vi "Check Status.vi"(8 "error in (no error)":errorcluster, 11 "Power Meter in":refnum<class "Power Meter.lvclass">) -> (0 "error out":errorcluster, 1 "Status":string, 2 "Ready?":bool, 3 "Power Meter out":refnum<class "Power Meter.lvclass">)   [LabVIEW 2009, in "Power Meter.lvclass"]
doc: "(Dynamic) Check if the instrument is powered on and update its member fields with the instrument's current status. Optionally return a text status message."
uses:
  Power Meter.lvclass
  Utility Classes/Readable/Readable.lvclass
  Power Meter.lvclass/Power Meter.ctl
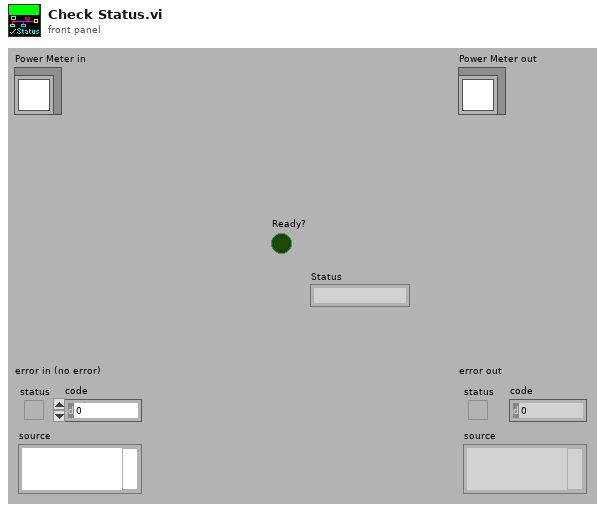
[diagram p1: front panel]
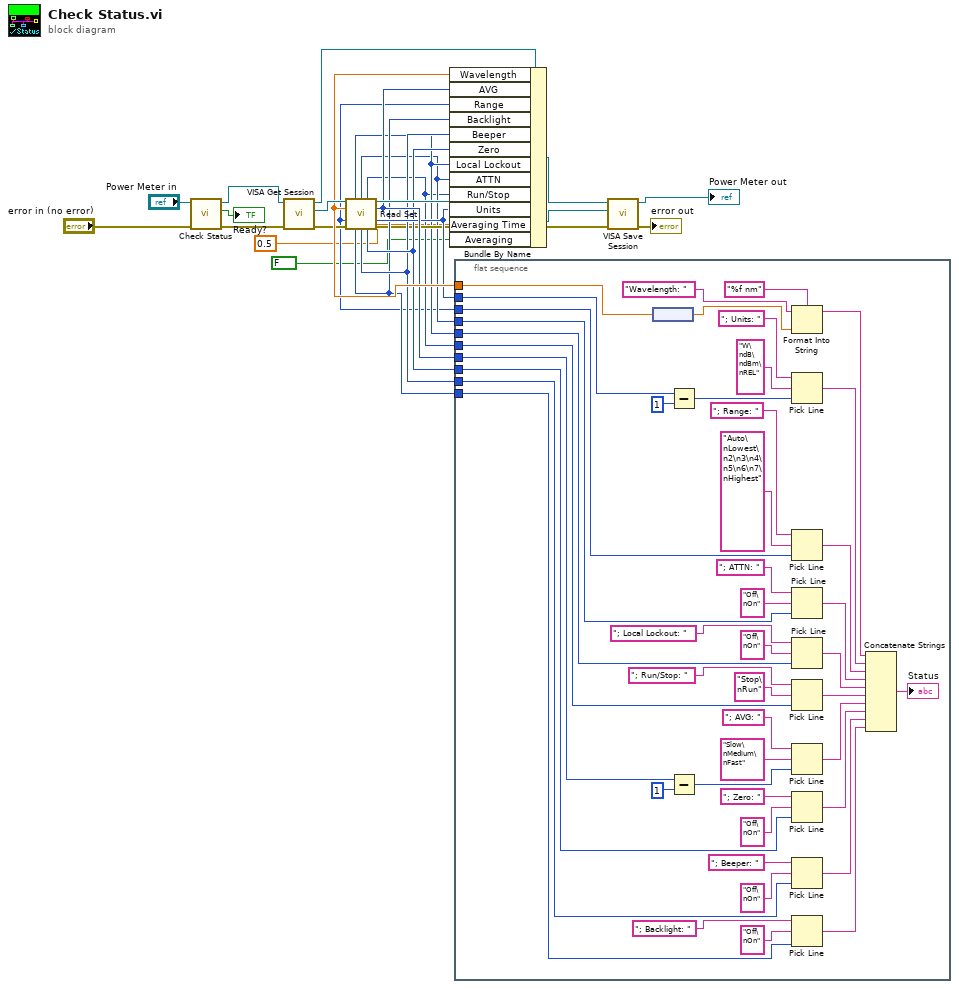
[diagram p0: block diagram]
diagram:
  n1 = call-parent "Check Status.vi"("error in (no error)"="error in (no error)", "Instrument in"="Power Meter in") -> ("error out"=w20:errorcluster, "Ready?"=→"Ready?":bool, "Instrument out"=w22:refnum<class "Power Meter.lvclass">)  [unwired: 6 in, 1 out]
  n2 = call-dynamic "VISA Get Session.vi"("error in (no error)"=w20, "Instrument.lvclass in"=w22) -> ("error out"=w8:errorcluster, "VISA Resource Name"=w16:refnum<visa-resource-name>, "Instrument.lvclass out"=w18:refnum<class "Power Meter.lvclass">)  [unwired: 7 out]
  n3 = call "Read Set.vi"("VISA resource name"=w16, "error in (no error)"=w8) -> ("Local Lockout"=w6:u32, "ATTN"=w5:u32, "Run/Stop"=w4:u32, "VISA resource name out"=w15:refnum<visa-resource-name>, "Wavelength (nnnn)"=w14:dbl[unit], "AVG"=w13:u32, "Range (1:8)"=w3:u32, "Units"=w12:u32, "Backlight"=w9:u32, "Beeper"=w10:u32, "Zero"=w11:u32, "error out"=w7:errorcluster)  [unwired: 2 in]
  n4 = Bundle By Name(cluster=w18, "Wavelength"=w14, "AVG"=w13, "Range"=w3, "Backlight"=w9, "Beeper"=w10, "Zero"=w11, "Local Lockout"=w6, "ATTN"=w5, "Run/Stop"=w4, "Units"=w12, "Averaging Time"=0.5, "Averaging"=FALSE) -> (w17:refnum<class "Power Meter.lvclass">)
  n5 = flat-sequence {
    tunnel: w12 -> [w63]
    tunnel: w14 -> [w59]
    tunnel: w5 -> [w57]
    tunnel: w3 -> [w53]
    tunnel: w6 -> [w49]
    tunnel: w4 -> [w45]
    tunnel: w13 -> [w41]
    tunnel: w11 -> [w35]
    tunnel: w10 -> [w31]
    tunnel: w9 -> [w27]
    frame #0 {
      n6 = node(w59) -> (w71:dbl)
      n7 = Subtract(x=w63, y=u32 1) -> (x-y=w61:u32)
      n8 = Subtract(x=w41, y=u32 1) -> (x-y=w39:u32)
      n9 = Format Into String(format string="%f nm", initial string="Wavelength: ", w71) -> (resulting string=w66:string)  [unwired: 1 in, 1 out]
      n10 = Pick Line(string ("")="; Units: ", multi-line string="W\ndB\ndBm\nREL", line index=w61) -> (output string=w65:string)
      n11 = Pick Line(string ("")="; Range: ", multi-line string="Auto\nLowest\n2\n3\n4\n5\n6\n7\nHighest", line index=w53) -> (output string=w52:string)
      n12 = Pick Line(string ("")="; ATTN: ", multi-line string="Off\nOn", line index=w57) -> (output string=w56:string)
      n13 = Pick Line(string ("")="; Local Lockout: ", multi-line string="Off\nOn", line index=w49) -> (output string=w48:string)
      n14 = Pick Line(string ("")="; Run/Stop: ", multi-line string="Stop\nRun", line index=w45) -> (output string=w44:string)
      n15 = Pick Line(string ("")="; AVG: ", multi-line string="Slow\nMedium\nFast", line index=w39) -> (output string=w38:string)
      n16 = Pick Line(string ("")="; Zero: ", multi-line string="Off\nOn", line index=w35) -> (output string=w34:string)
      n17 = Pick Line(string ("")="; Beeper: ", multi-line string="Off\nOn", line index=w31) -> (output string=w30:string)
      n18 = Pick Line(string ("")="; Backlight: ", multi-line string="Off\nOn", line index=w27) -> (output string=w26:string)
      n19 = Concatenate Strings(w66, w65, w52, w56, w48, w44, w38, w34, w30, w26) -> (→"Status":string)
    }
  }
  n20 = call-dynamic "VISA Save Session.vi"("error in (no error)"=w7, "VISA Resource Name"=w15, "Instrument.lvclass in"=w17) -> ("error out"=→"error out":errorcluster, "Instrument.lvclass out"=→"Power Meter out":refnum<class "Power Meter.lvclass">)  [unwired: 7 out]
